vi "AccurusCtrlDemo.vi"() -> ()   [LabVIEW 2010]
uses:
  <vilib>/rvi/interface/nirviReadWriteControl/nirviReadWriteControl.xnode
  FPGA Bitfiles/IRISSControl_FPGATarget_QuadCtr2_FdSaI9MfFZo.lvbitx
  IRISS_FPGA_IO.vi
  <vilib>/rvi/interface/nirviOpenFPGA/nirviOpenFPGA.xnode
  <vilib>/rvi/interface/nirviCloseFPGA/nirviCloseFPGA.xnode
  <vilib>/rvi/interface/nirviMethod/nirviMethod.xnode
panel:
  in  "stop":bool
  in  "Aspiration Pressure [mmHg]":i16(slide) scale=0.0..600.0
  out "Error(s) Out on Program End":errorcluster
  in  "Accurus Ctrl Cluster":T1={"Stop Vacuum"=TRUE, "Vacuum Force"=0, "Max Limit [mmHg]"=600.0, "Slide in"=0, "Irrigation?"=TRUE} {"Slide in" scale=0.0..78.0; "Vacuum Force" min=0 max=78}
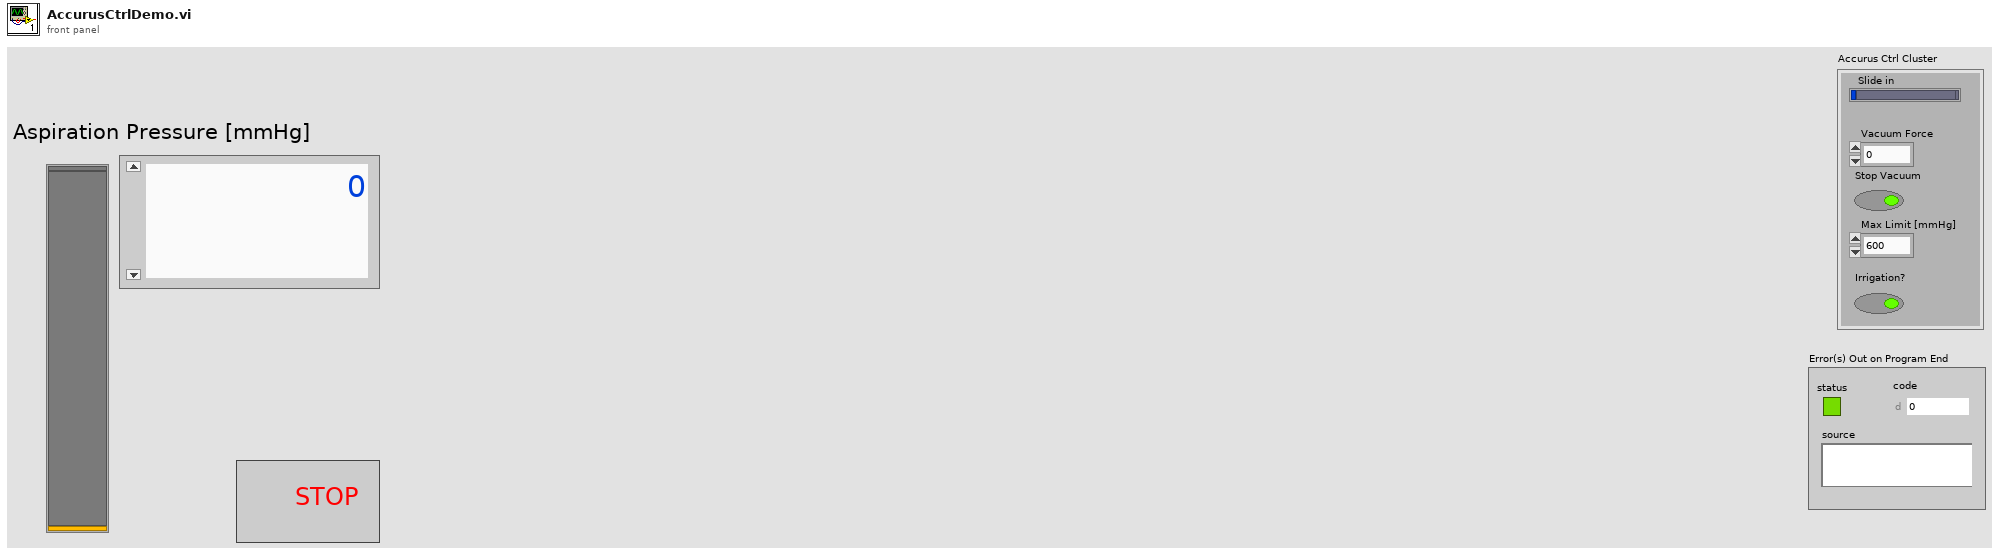
[diagram p1: front panel]
types:
  T1 = cluster{"Stop Vacuum":bool, "Vacuum Force":i8, "Max Limit [mmHg]":dbl, "Slide in":i8, "Irrigation?":bool}
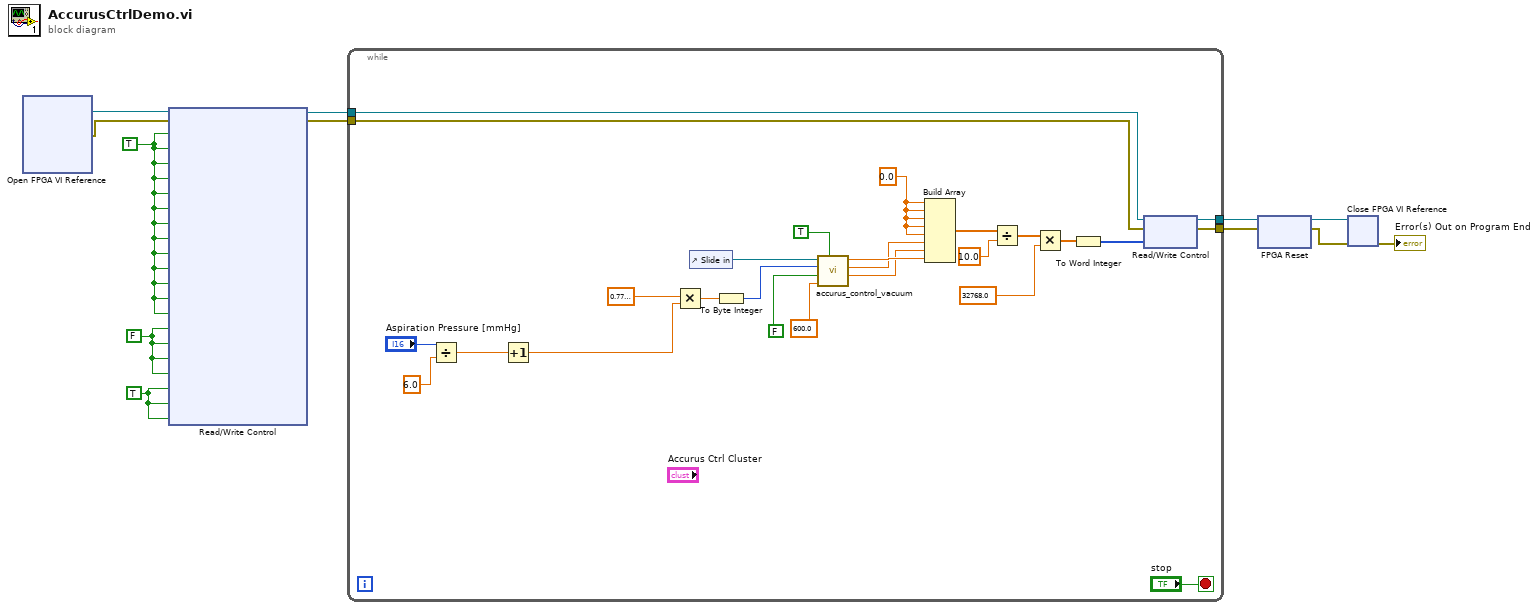
[diagram p0: block diagram]
diagram:
  w11 = TRUE ("Conn0/DIO12 Button 1")
  w10 = FALSE ("Reset")
  w12 = TRUE ("Reset")
  n1 = xnode "Open FPGA VI Reference"() -> ("FPGA VI Reference Out"=w9:refnum<k20>, "error out"=w8:errorcluster)  [unwired: 2 in]
  n2 = xnode "Read/Write Control"("FPGA VI Reference In"=w9, "error in"=w8, "Reset 1"=w12, "Reset 3"=w12, "Reset 9"=w12, "Reset 10"=w12, "Reset 11"=w12, "Reset 12"=w12, "Reset 13"=w12, "Reset 14"=w12, "Reset 15"=w12, "Reset 16"=w12, "Reset 17"=w12, "Reset C1-1"=w12, "Reset C1-4"=w12, "INHB X"=w10, "INHB Y"=w10, "INHB Z"=w10, "INHB OCT Mot"=w10, "Conn0/DIO12 Button 1"=w11, "Conn0/DIO13 Button 2"=w11, "Conn0/DIO15 Button 4"=w11) -> ("FPGA VI Reference Out"=w3:refnum<k20>, "error out"=w2:errorcluster)
  n3 = while {
    tunnel: [w24] -> w4
    tunnel: w3 -> [w23]
    tunnel: w2 -> [w22]
    tunnel: [w21] -> w1
    stop <- "stop" stop-if-true
    w31 = 0.0
    n4 = Divide(x="Aspiration Pressure [mmHg]", y=sgl 6.0) -> (x/y=w14:sgl)
    n5 = Increment(x=w14) -> (x+1=w13:sgl)
    n6 = Multiply(x=sgl 0.78 ("y"), y=w13) -> (x*y=w20:sgl)
    n7 = control-ref of="Slide in"() -> (w34:refnum<vi>)
    n8 = To Byte Integer(number=w20) -> (8bit integer=w19:i8)
    n9 = call "accurus_control_vacuum.vi"("Irrigate?"=TRUE, "Max Limit [mmHg]"=600.0, "stop"=FALSE, "vacuum force"=w19, "Slide in"=w34) -> ("f"=w25:dbl, "f 2"=w26:dbl, "f 3"=w35:dbl)  [unwired: 1 in, 3 out]
    n10 = Build Array(w31, w31, w31, w31, w31, w26, w25, w35) -> (w38:dbl[])
    n11 = Divide(x=w38, y=10.0) -> (x/y=w36:dbl[])
    n12 = Multiply(x=w36, y=32768.0) -> (x*y=w33:dbl[])
    n13 = To Word Integer(number=w33) -> (16bit integer=w32:i16[])
    n14 = xnode "Read/Write Control"("FPGA VI Reference In"=w23, "error in"=w22, "AO"=w32) -> ("FPGA VI Reference Out"=w24:refnum<k20>, "error out"=w21:errorcluster)
  }
  n15 = xnode "FPGA Reset"("FPGA VI Reference In"=w4, "error in"=w1) -> ("FPGA VI Reference Out"=w7:refnum<k20>, "error out"=w6:errorcluster)
  n16 = xnode "Close FPGA VI Reference"("FPGA VI Reference In"=w7, "error in"=w6) -> ("error out"=→"Error(s) Out on Program End":errorcluster)
